vi "FBClassVI.vi"(8 "String2":string=" SMALLcaps", 11 "String1":string="largecaps") -> (3 "String Output":string="LARGECAPS smallcaps")   [LabVIEW 2023, in "FBClass.lvclass"]
doc: "Output = String1 (in largecaps) + String2 (in smallcaps)"
uses:
  FBClass.lvclass
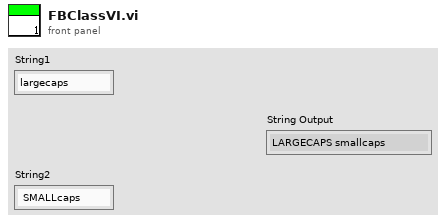
[diagram p1: front panel]
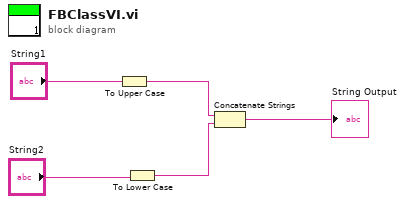
[diagram p0: block diagram]
diagram:
  n1 = To Upper Case(1:"String1") -> (0:w3:string)
  n2 = To Lower Case(string="String2") -> (all lower case string=w2:string)
  n3 = Concatenate Strings(w3, w2) -> (→"String Output":string)
